vi "Compute Motor Model Values.vi"(9 "Breaker Size":dbl[unit]=0.7, 11 "Motor Coefficients":T2={"Stall Torque"=0.71, "Stall Current"=134.0, "Free Speed"=18730.0, "Free Speed Current"=0.7, "Name"=""}) -> (3 "Motor Model Values":T1 {"Free Current" format="%#_3p"; "Breaker Size" format="%#_3p"; "Kv" format="%#_3p"; "R" format="%#_3p"; "Kt" format="%#_3p"})   [LabVIEW 2020]
uses:
  Motor Coefficients.ctl
  Modeling/Motor Operating Values.ctl
panel:
  # "rpm"
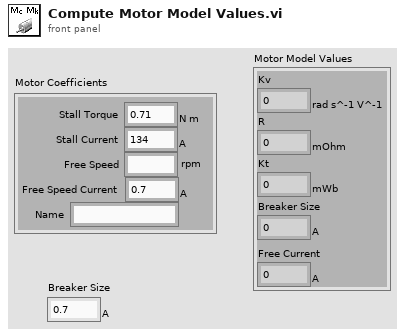
[diagram p1: front panel]
types:
  T1 = typedef "Motor Operating Values.ctl" = cluster{"Kv":dbl[unit], "R":dbl[unit], "Kt":dbl[unit], "Breaker Size":dbl[unit], "Free Current":dbl[unit]}
  T2 = typedef "Motor Coefficients.ctl" = cluster{"Stall Torque":dbl[unit], "Stall Current":dbl[unit], "Free Speed":dbl, "Free Speed Current":dbl[unit], "Name":string}
  T3 = cluster{dbl[unit], dbl[unit], dbl[unit], "Breaker Size":dbl[unit], "Free Speed Current":dbl[unit]}
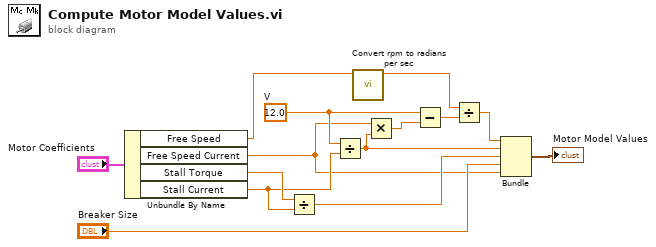
[diagram p0: block diagram]
diagram:
  w11 = dbl[unit] 12.0  # V
  n1 = Unbundle By Name("Motor Coefficients") -> ("Free Speed"=w5:dbl, "Free Speed Current"=w1:dbl[unit], "Stall Torque"=w14:dbl[unit], "Stall Current"=w2:dbl[unit])
  n2 = Divide(x=w14, y=w2) -> (x/y=w6:dbl[unit])
  n3 = Divide(x=w11, y=w2) -> (x/y=w7:dbl[unit])
  n4 = call "Convert rpm to radians per sec.vi"("motor speed (rpm)"=w5) -> ("speed rps"=w4:dbl[unit])  [unwired: 10 in]
  n5 = Multiply(x=w1, y=w7) -> (x*y=w10:dbl[unit])
  n6 = Subtract(x=w11, y=w10) -> (x-y=w12:dbl[unit])
  n7 = Divide(x=w4, y=w12) -> (x/y=w8:dbl[unit])
  n8 = Bundle(w8, w7, w6, "Breaker Size"="Breaker Size", "Free Speed Current"=w1) -> (→"Motor Model Values":T3)  [unwired: 1 in]
